vi "Process.vi"(8 "error in":errorcluster, 11 "Instrument.OxfordVRM UI.lvclass":refnum<class "Instrument.OxfordVRM UI.lvclass">) -> (0 "error out":errorcluster, 3 "Instrument.OxfordVRM UI.lvclass":refnum<class "Instrument.OxfordVRM UI.lvclass">)   [LabVIEW 2019, in "Instrument.OxfordVRM UI.lvclass"]
doc: "---------------------------------------------------------------\nJKI State Machine Objects™\nhttp://jki.net/state-machine-objects/\nCopyright (C) 2005-2015, JKI <info@jki.net>\nALL RIGHTS RESERVEDJKI State Machine Objects (SMO) 1.0.0.5\nJKI - JKI\nCopyright (c) 2016, JKI"
uses:
  Instrument.OxfordVRM UI.lvclass
  <vilib>/JKI/JKI SMO/SMO/SMO.lvclass
  <vilib>/JKI/JKI SMO/SMO.UI/SMO.UI.lvclass
  <userlib>/LevyLab/Instrument Framework/Instrument/Instrument.lvclass
  Instrument.OxfordVRM/Typedefs/getAll.ctl
  Instrument.OxfordVRM/Instrument.OxfordVRM.lvclass
  <userlib>/LevyLab/Instrument Framework/Instrument UI/Instrument UI.lvclass
  Instrument.OxfordVRM/Typedefs/VRM Magnet Axis--Enum.ctl
  C:/Program Files (x86)/National Instruments/LabVIEW 2019/user.lib/LevyLab/Instrument Framework/Instrument Types/Cryostat/Instrument.Cryostat.lvclass
  C:/Program Files (x86)/National Instruments/LabVIEW 2019/user.lib/LevyLab/Instrument Framework/Instrument/Instrument.lvclass
  C:/Program Files (x86)/National Instruments/LabVIEW 2019/vi.lib/JKI/JKI SMO/SMO/SMO.lvclass
  C:/Program Files (x86)/National Instruments/LabVIEW 2019/user.lib/LevyLab/Instrument Framework/Instrument UI/Instrument UI.lvclass
  C:/Program Files (x86)/National Instruments/LabVIEW 2019/vi.lib/JKI/JKI SMO/SMO.UI/SMO.UI.lvclass
panel:
  in  "Rate (T/min)":dbl[](array[numeric])=[0.0]
  out "Status":string[](array[string])
  in  "Coordinates":enum16{"XYZ", "Sph"}(ring)
  out "Set Rate (T/min)":dbl[](array[numeric])
  in  "Target (T)":dbl[](array[numeric])=[0.0, 0.0, 0.0]
  out "Setpoint (T)":dbl[](array[numeric])
  out "Field (T)":dbl[](array[numeric])
  out "XY Graph":cluster{dbl[], dbl[]}[](graph)
  out "XZ Graph":cluster{dbl[], dbl[]}[](graph)
  out "Voltage Meter 6":dbl(knob) scale=-10.0..10.0
  out "Voltage Meter 5":dbl(knob) scale=-10.0..10.0
  out "Voltage Meter 4":dbl(knob) scale=-10.0..10.0
  out "Voltage Meter 3":dbl(knob) scale=-10.0..10.0
  out "Voltage Meter 2":dbl(knob) scale=-10.0..10.0
  out "Current Meter 6":dbl(knob) scale=-120.0..120.0
  out "Current Meter 5":dbl(knob) scale=-120.0..120.0
  out "Current Meter 4":dbl(knob) scale=-120.0..120.0
  out "Current Meter 3":dbl(knob) scale=-120.0..120.0
  out "Current Meter 2":dbl(knob) scale=-120.0..120.0
  out "Voltage Meter 1":dbl(knob) scale=-10.0..10.0
  out "Current Meter 1":dbl(knob) scale=-120.0..120.0
  out "System Time (HH:MM:SS)":dbl=165.3592643737793 format="%<%I:%M:%S %p>T"
  out "ETA":dbl=3660699600.0 format="%<%I:%M:%S %p %m/%d/%Y>T"
  out "version":string="v20/10/28"
  in  "Window Maximize":bool
  in  "Window Minimize":bool
  in  "Hold":bool
  in  "To Set":bool
  in  "Export":bool
  in  "To Zero":bool
  in  "Clamp":bool
  out "Magnet Status 2":string="Status: Clamped"
  in  "Power":bool
  # "Status"
  # "x"
  # "Actions"
  # "Targets"
  # "Status"
  # "x"
  # "y"
  # "X \t\t\nCurrent (A)\tField (T)\t    Rate (T/')\n0  - 30 \t   0    - 0.6 \t  0.06\n30 - 42\t    0.6  - 0.85\t  0.048\n42 - 60\t    0.85 - 1.2\t   0.042\n60 - 80\t    1.2  - 1.6\t   0.036\n80 - 99\t    1.6  - 2.0\t   0.024\n\nY \t\t\nCurrent (A)\tField (T)\t    Rate (T/')\n0  - 30\t    0    - 0.6\t   0.048\n30 - 35\t    0.6  - 0.69\t  0.035\n35 - 45\t    0.69 - 0.89\t  0.03\n45 - 60\t    0.89 - 1.2\t   0.024\n60 - 80\t    1.2  - 1.58\t  0.018\n80 - 101\t   1.58 - 2\t     0.01\n\nZ \t\t\nCurrent (A)\tField (T)\t    Rate (T/')\n0  - 30\t    0    - 2.6    0.26\n30 - 60\t    2.6  - 5.3\t   0.21\n60 - 80\t    5.3  - 7.1\t   0.16\n80 - 90\t    7.1  - 8\t     0.13\n90 - 101\t   8    - 9\t     0.1\n\n2 OR MORE AXES\n0.005 T/min"
  # "z"
  # "z"
  # "PS Status"
  # "y"
  # "SMO UI Template"
  # "For instructions on how to use the JKI State Machine Objects, examples and video tutorials, visit:\nhttp://jki.net/state-machine-objects/\n\nJKI State Machine Objects™\nhttp://jki.net/state-machine-objects/\nCopyright (C) 2005-2015, JKI <info@jki.net>\nALL RIGHTS RESERVED"
  # "PSU 6 Voltage (V)"
  # "PSU 5 Voltage (V)"
  # "PSU 4 Voltage (V)"
  # "PSU 3 Voltage (V)"
  # "PSU 2 Voltage (V)"
  # "PSU 6 Current (A)"
  # "PSU 5 Current (A)"
  # "PSU 4 Current (A)"
  # "PSU 3 Current (A)"
  # "PSU 2 Current (A)"
  # "PSU 1 Voltage (V)"
  # "PSU 1 Current (A)"
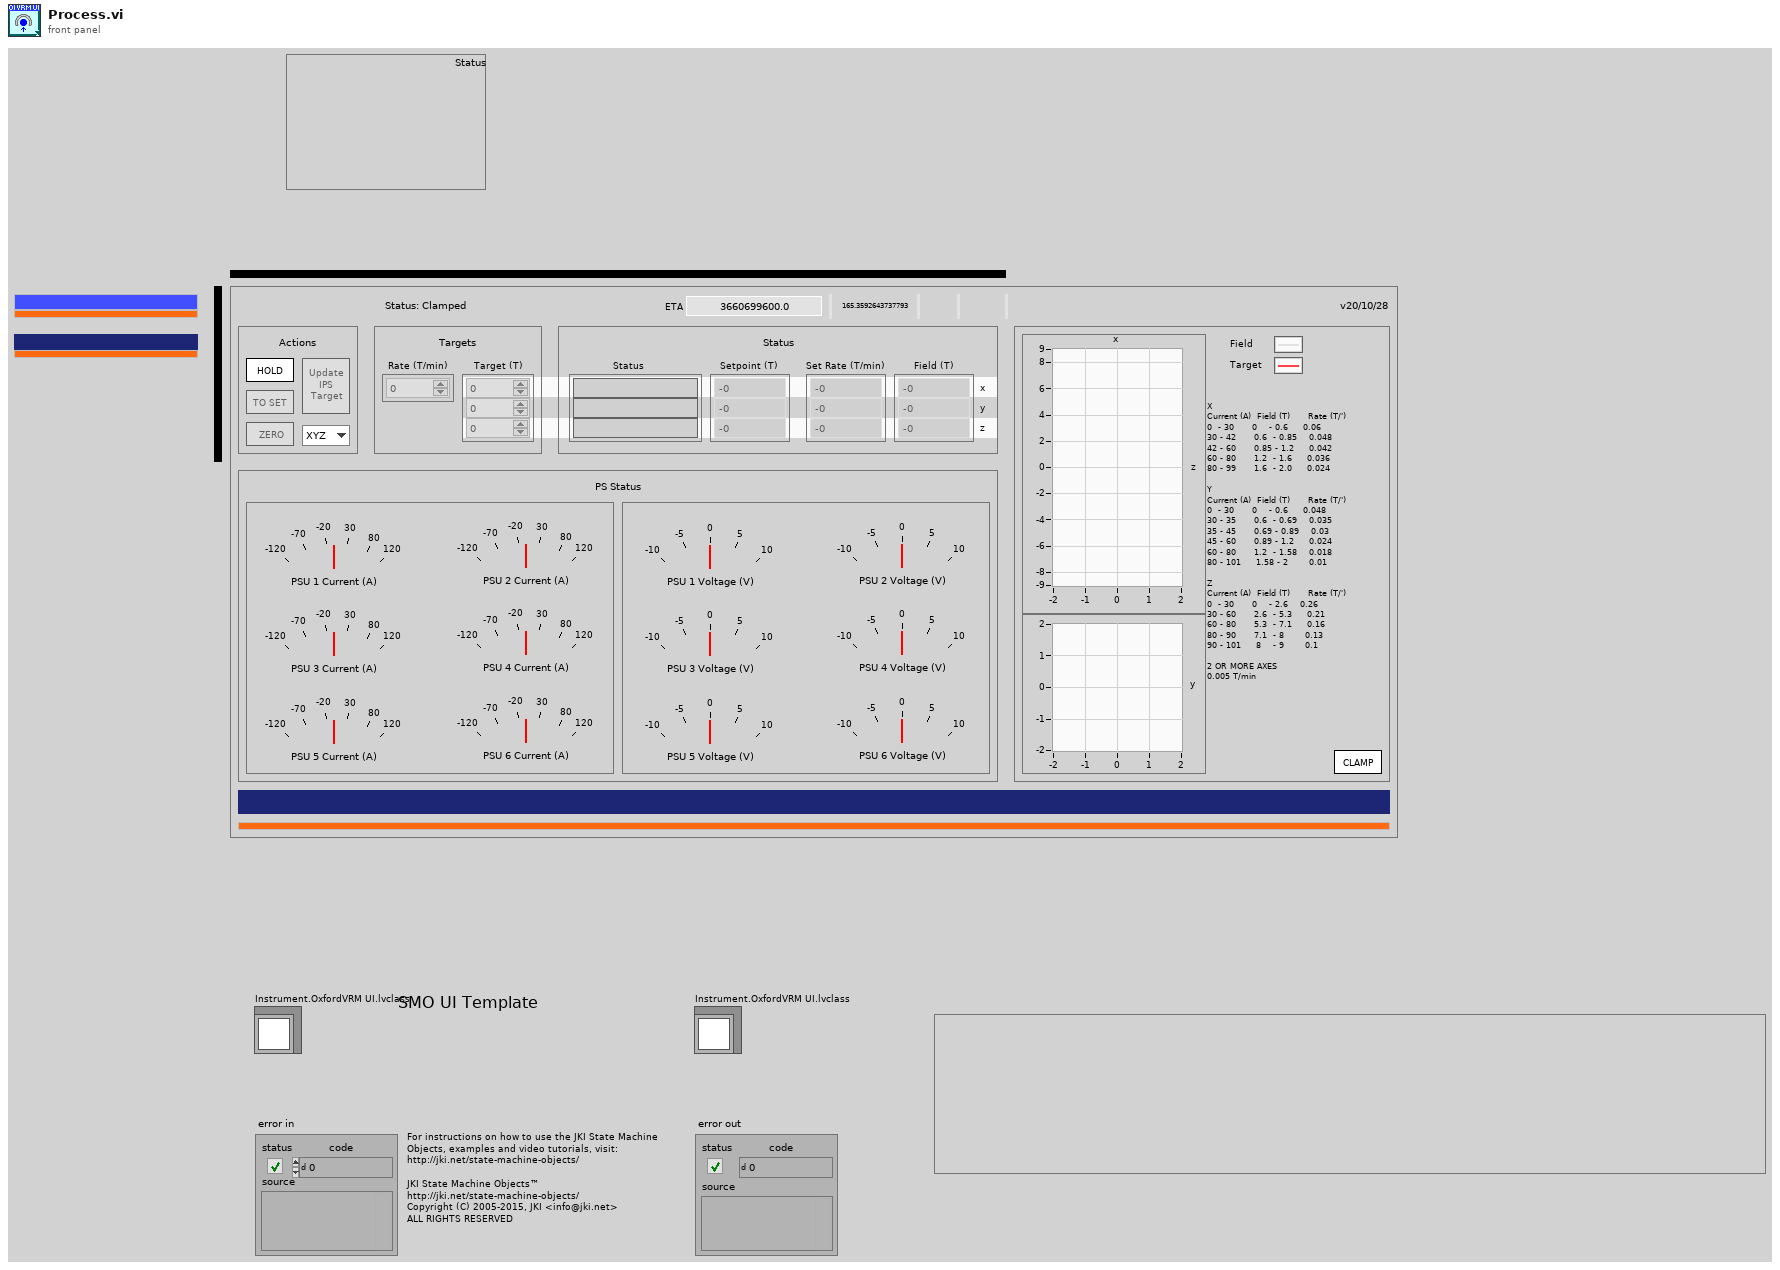
[diagram p1: front panel]
types:
  T1 = typedef "Instrument.OxfordVRM.lvclass/getAll.ctl" = cluster{"Field":dbl[], "Target Field":dbl[], "Target Field Rate":dbl[], "PSU Current":dbl[], "PSU Voltage":dbl[], "Status":string[]}
  T2 = enum32{"invalid app kind", "Development System", "Run Time System", "Student Edition", "Embedded LabVIEW", "Evaluation", "Custom"}
  T3 = enum32{"Invalid", "Standard", "Closed", "Hidden", "Minimized", "Maximized"}
  T4 = typedef "Instrument.OxfordVRM.lvclass/VRM Magnet Axis--Enum.ctl" = enum16{"Z", "X", "Y", "ALL"}
  T5 = cluster{"Core":cluster{"Current VI Reference":refnum<vi>, "Close Panel on Exit?":bool, "error":errorcluster}, "Instrument UI":refnum<class "Instrument.OxfordVRM UI.lvclass">, "Instrument":refnum<class "Instrument.OxfordVRM.lvclass">, "getAll":T1, "Response":string, "config":variant, "Setpoint (XYZ)":dbl[]}
  T6 = typedef "Instrument.OxfordVRM.lvclass/PublicEvents--Instrument.Oxford1820.ProcessStatus.ctl" = string
  T7 = cluster{"Current VI Reference":refnum<vi>, "Close Panel on Exit?":bool, "error":errorcluster}
  T8 = typedef "LVRectTypeDef.ctl" = cluster{"Left":i16, "Top":i16, "Right":i16, "Bottom":i16}
  T9 = typedef "smo.lvlib/SMO.lvclass/Protected Events.ctl" = cluster{"StopProcesses":refnum<user-event>, "AbortProcesses":refnum<user-event>, "Config Changed":refnum<user-event>, "Dependency":refnum<user-event>}
  T10 = typedef "Instrument.lvlib/Instrument.lvclass/PublicEvents--Cluster.ctl" = cluster{"MessageFromProcess":refnum<user-event>}
  T11 = typedef "Instrument.OxfordVRM.lvclass/PublicEvents--Cluster.ctl" = cluster{"ProcessStatus":refnum<user-event>}
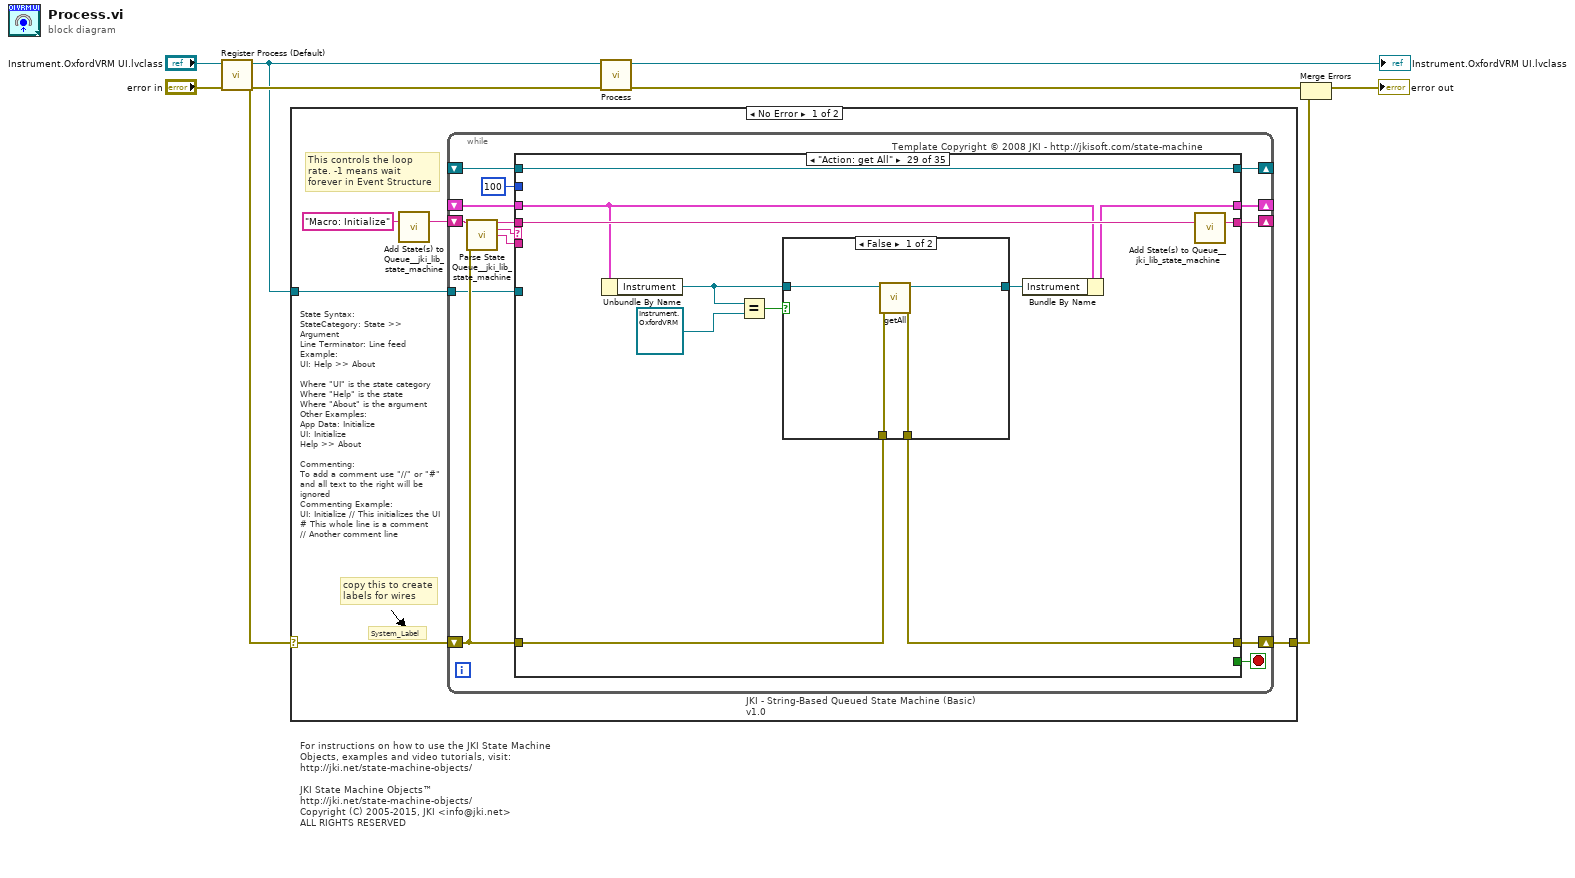
[diagram p0: block diagram]
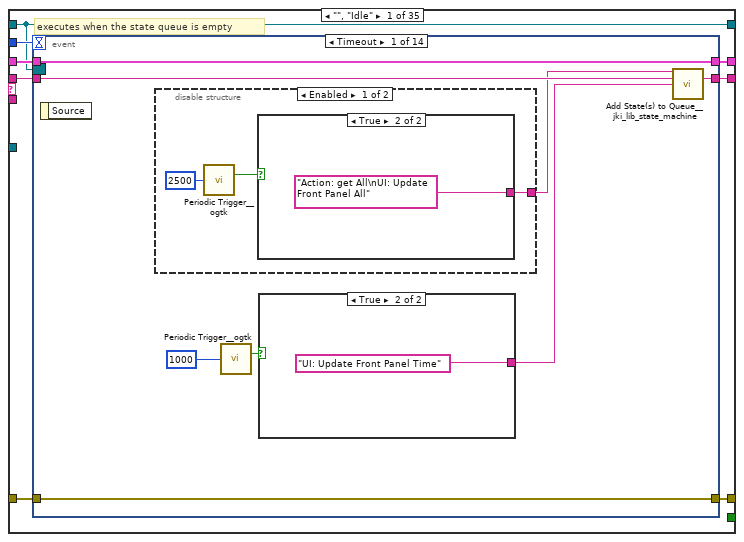
[diagram p2: hidden frame]
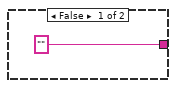
[diagram p3: hidden frame]
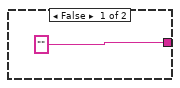
[diagram p4: hidden frame]
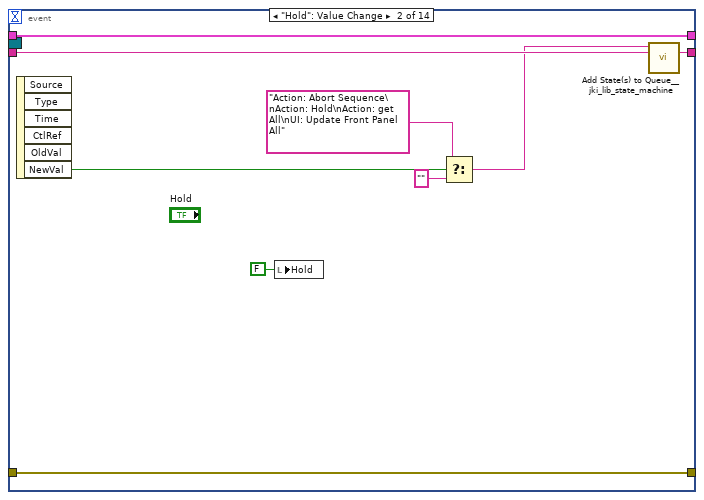
[diagram p6: hidden frame]
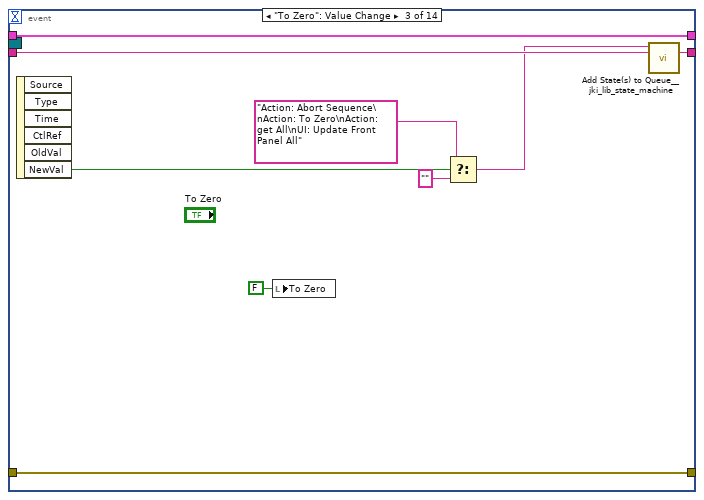
[diagram p7: hidden frame]
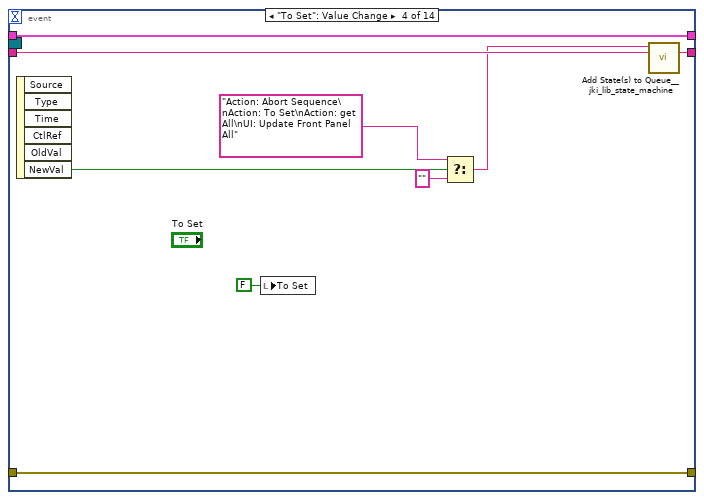
[diagram p8: hidden frame]
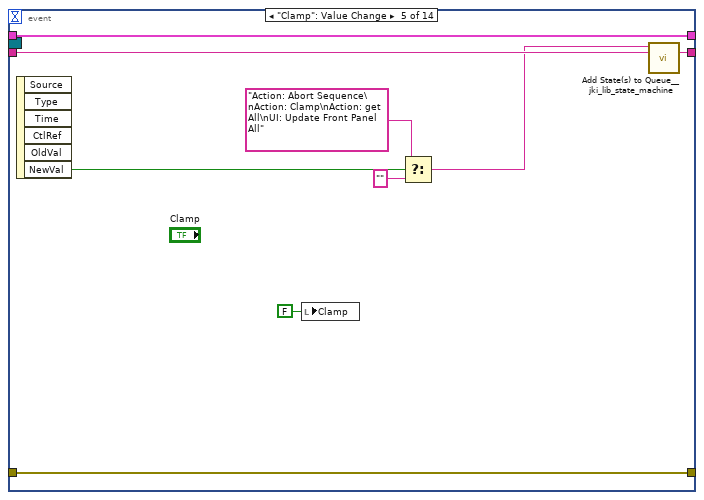
[diagram p9: hidden frame]
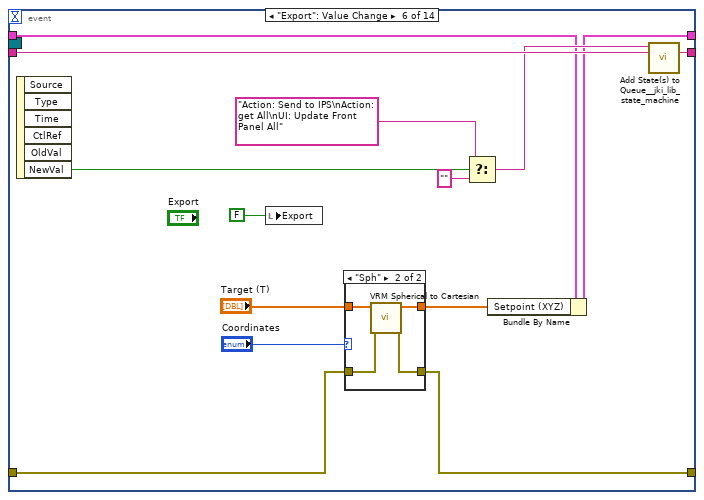
[diagram p10: hidden frame]
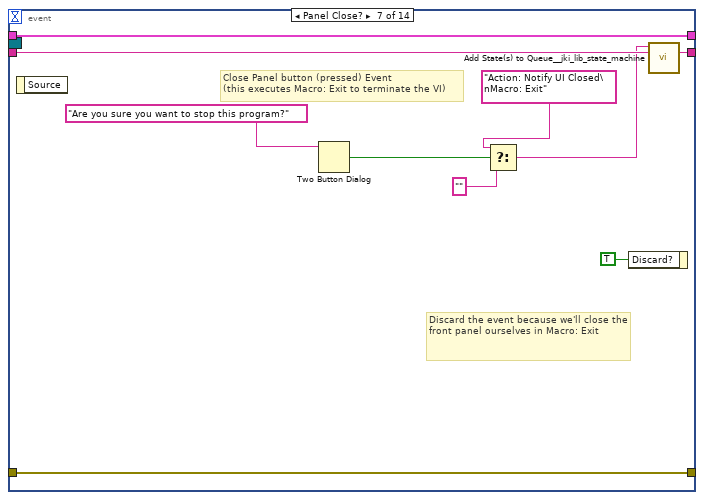
[diagram p12: hidden frame]
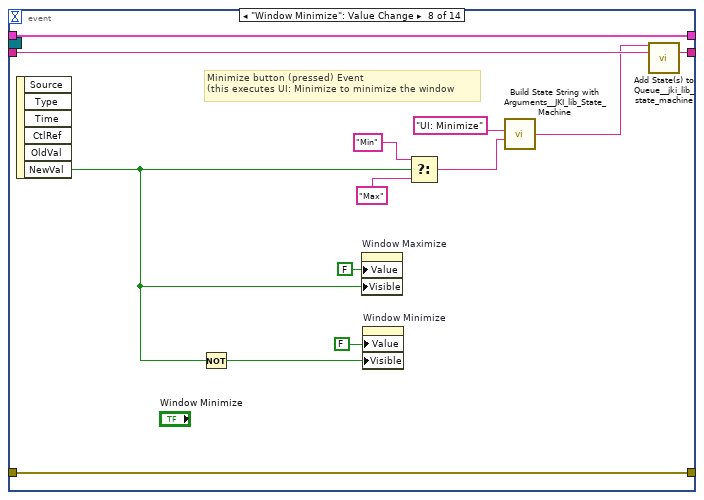
[diagram p13: hidden frame]
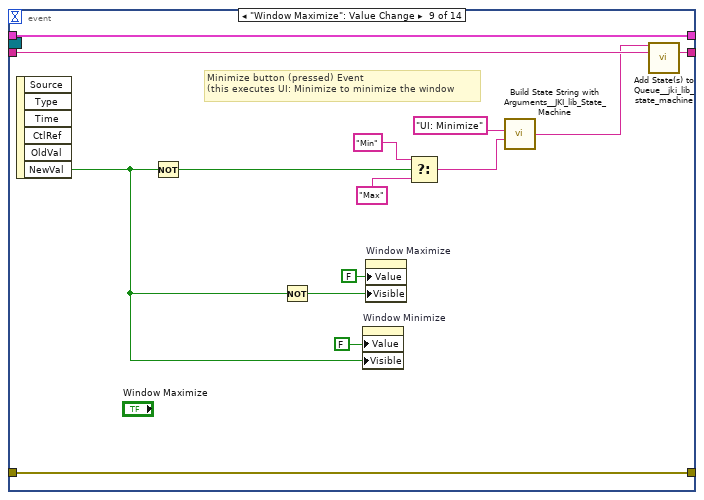
[diagram p14: hidden frame]
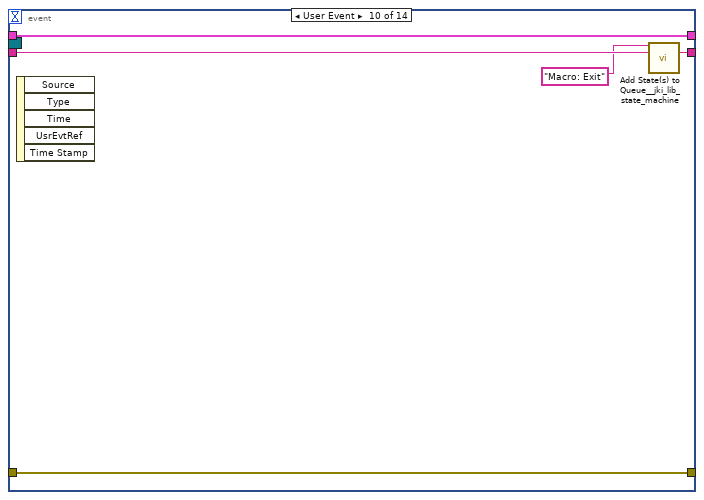
[diagram p15: hidden frame]
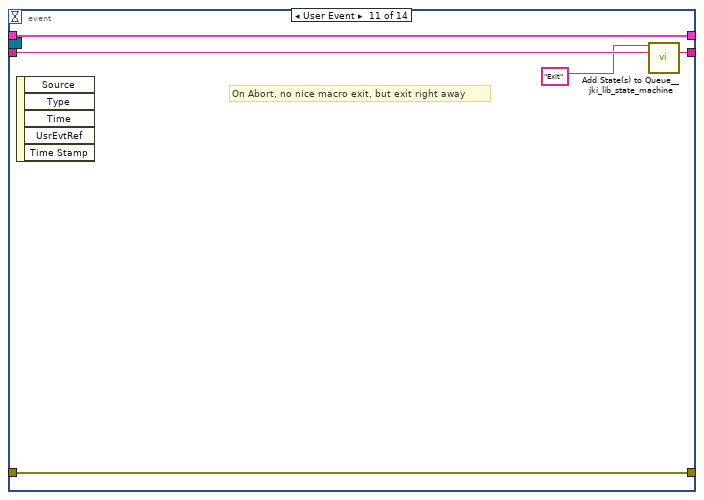
[diagram p16: hidden frame]
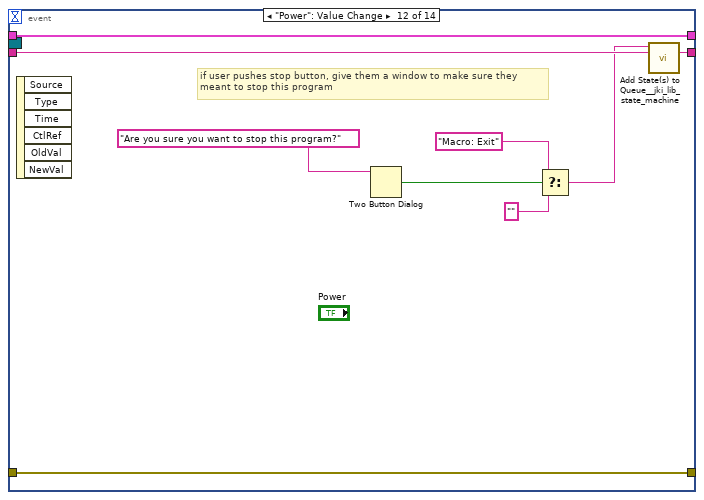
[diagram p17: hidden frame]
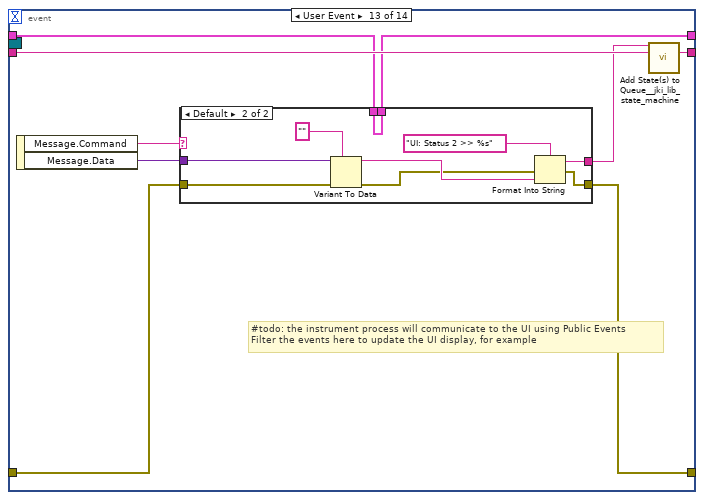
[diagram p18: hidden frame]
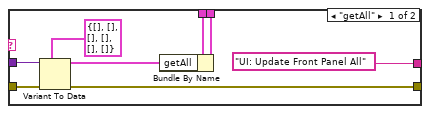
[diagram p19: hidden frame]
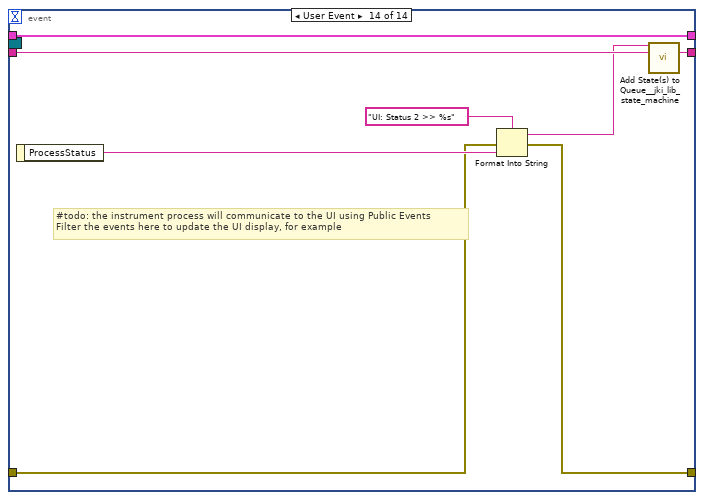
[diagram p20: hidden frame]
diagram:
  # "For instructions on how to use the JKI State Machine Objects, examples and video tutorials, visit:\nhttp://jki.net/state-machine-objects/\n\nJKI State Machine Objects™\nhttp://jki.net/state-machine-objects/\nCopyright (C) 2005-2015, JKI <info@jki.net>\nALL RIGHTS RESERVED"
  n1 = call <vilib>:"Register Process (Default).vi"("error in (no error)"="error in", "SMO"="Instrument.OxfordVRM UI.lvclass") -> ("error out"=w5:errorcluster, "SelfRef"=w4:refnum<class "Instrument.OxfordVRM UI.lvclass">)  [unwired: 8 in]
  n2 = case shown="No Error" w5 {
    selector: w5 -> [w10 w612]
    tunnel: w4 -> [w11 _]
    tunnel: [w9 w612] -> w1
    frame No Error {
      # "State Syntax:\nStateCategory: State >> Argument\nLine Terminator: Line feed\nExample:\nUI: Help >> About\n\nWhere \"UI\" is the state category\nWhere \"Help\" is the state\nWhere \"About\" is the argument\nOther Examples:\nApp Data: Initialize\nUI: Initialize\nHelp >> About\n\nCommenting:\nTo add a comment use \"//\" or \"#\" and all text to the right will be ignored\nCommenting Example:\nUI: Initialize // This initializes the UI\n# This whole line is a comment\n// Another comment line"
      # "copy this to create labels for wires"
      # "This controls the loop rate. -1 means wait forever in Event Structure"
      # "System_Label"
      n3 = call <vilib>:"Add State(s) to Queue__jki_lib_state_machine.vi"("State(s) in (\"\")"="Macro: Initialize") -> ("States Out"=w13:string)  [unwired: 14 in]
      n4 = while "JKI - String-Based Queued State Machine (Basic) v1.0" {
        shift-right: [w20] -> _
        shift-left: _ -> [w19]
        shift-right: [w23] -> w9
        shift-left: w10 -> [w17]
        shift-right: [w22] -> _
        shift-left: w13 -> [w24]
        tunnel: w11 -> [w16]
        shift-right: [w15] -> _
        shift-left: _ -> [w14]
        stop <- w21 stop-if-true
        # "Template Copyright © 2008 JKI - http://jkisoft.com/state-machine"
        n5 = call <vilib>:"Parse State Queue__jki_lib_state_machine.vi"("State Queue"=w24, "Error In (no error)"=w17) -> ("Remaining States"=w26:string, "Current State"=w27:string, "Arguments"=w25:string)  [unwired: 11 in]
        n6 = case shown="\"Action: get All\"" w27 {
          selector: w27 -> [_ _ w203 _ _ _ _ _ _ _ _ _ _ _ _ _ _ _ _ _ _ _ _ _ _ _ _ _ _ _ _ _ _ _ _]
          tunnel: w26 -> [w35 w201 w207 w226 w240 w246 w251 w270 w277 w282 w296 w327 w348 w362 w369 w385 w419 w445 w454 w468 w473 w484 w491 w496 w512 w518 w525 w532 w543 w558 w568 w578 w588 w598 w611]
          tunnel: w25 -> [_ _ _ _ _ _ _ _ _ _ _ _ _ w357 w363 w379 w420 _ _ _ _ _ _ _ _ _ _ _ _ _ _ _ _ _ _]
          tunnel: w19 -> [w33 w198 w205 w217 w228 w242 w248 _ w272 w279 w294 w324 w342 w359 w367 w381 w418 w442 w450 w459 w470 w481 w486 w493 w510 w516 w521 w528 w536 w550 w559 w569 w579 w590 w600]
          tunnel: [w32 w199 w209 w223 w233 w241 w249 w254 w273 w280 w291 w323 w341 w360 w364 w382 w413 w443 w452 w466 w471 w475 w487 w494 w506 w513 w522 w526 w538 w553 w565 w575 w585 w595 w606] -> w23
          tunnel: w17 -> [w31 w199 w208 w223 w229 _ w249 w267 w274 w280 w292 w297 w341 w360 w365 w383 w414 w443 w452 w466 w471 w476 w488 w494 w501 w514 w522 w527 w539 w554 w562 w572 w582 w592 w607]
          tunnel: [w34 w200 w206 w225 w239 w245 w250 w269 w276 w281 w295 w326 w347 w361 w368 w384 w424 w444 w453 w467 w472 w483 w490 w495 w511 w517 w524 w531 w542 w557 w567 w577 w587 w597 w610] -> w22
          tunnel: [_ _ _ _ _ TRUE _ _ _ _ _ _ _ _ _ _ _ _ _ _ _ _ _ _ _ _ _ _ _ _ _ _ _ _ _] -> w21
          tunnel: [w30 w198 w205 w224 w231 w242 w248 w268 w272 w279 w294 w324 w342 w359 w367 w381 w418 w442 w450 w459 w470 w481 w486 w493 w510 w516 w520 w528 w540 w552 w561 w571 w581 w591 w601] -> w20
          tunnel: 100 ("Timeout") -> [w29 _ _ _ _ _ _ _ _ _ _ _ _ _ _ _ _ _ _ _ _ _ _ _ _ _ _ _ _ _ _ _ _ _ _]
          tunnel: w16 -> [_ _ _ _ _ _ _ w261 _ _ _ _ _ _ _ _ _ _ _ _ _ _ _ _ _ _ _ _ _ _ _ _ _ _ _]
          tunnel: [w28 w197 w202 w214 w238 w243 w247 w265 w271 w278 w293 w325 w346 w358 w366 w378 w423 w441 w451 w460 w469 w482 w489 w492 w509 w515 w523 w530 w541 w556 w566 w576 w586 w596 w609] -> w15
          tunnel: w14 -> [w28 w197 w202 w214 w238 w243 w247 w265 w271 w278 w293 w325 w346 w358 w366 w378 w423 w441 w451 w460 w469 w482 w489 w492 _ w515 w523 w530 w541 w556 w566 w576 w586 w596 w609]
          frame "", "Idle" {
            # "executes when the state queue is empty"
            n7 = event shown="[0] Timeout" {
              selector: w28 -> [_ _ _ _ _ _ _ _ _ _ _ _ _ _]
              dyn-events: _ -> [_ _ _ _ _ _ _ _ _ _ _ _ _ _]
              timeout: w29 -> [_ _ _ _ _ _ _ _ _ _ _ _ _ _]
              tunnel: w35 -> [w43 w59 w68 w77 w86 w100 w116 w129 w143 w148 w153 w162 w171 w196]
              tunnel: [w42 w58 w67 w76 w85 w99 w115 w128 w142 w147 w152 w161 w170 w195] -> w34
              tunnel: w33 -> [w39 w56 w65 w74 w83 w93 w113 w127 w141 w145 w150 w159 w169 w190]
              tunnel: [w41 w57 w66 w75 w84 w87 w112 w126 w140 w146 w151 w160 w165 w189] -> w32
              tunnel: w31 -> [w41 w57 w66 w75 w84 w88 w112 w126 w140 w146 w151 w160 w166 w191]
              tunnel: [w39 w56 w65 w74 w83 w92 w113 w127 w141 w145 w150 w159 w168 w190] -> w30
              event Timeout {
                n8 = event-data() -> ()  [unwired: 1 in, 1 out]
                n9 = disable-structure shown="Enabled" {
                  disable-tunnel: [w46 _] -> w40
                  frame Enabled {
                    n10 = call <userlib>:"Periodic Trigger__ogtk.vi"("time (ms)"=u32 2500 ("update time (ms)")) -> ("Triggered"=w48:bool)  [unwired: 12 in, 2 out]
                    n11 = case shown="True" w48 {
                      tunnel: ["" "Action: get All\nUI: Update Front Panel All"] -> w46
                      frame False {
                      }
                      frame True {
                      }
                    }
                  }
                  frame Disabled {
                  }
                }
                n12 = call <userlib>:"Periodic Trigger__ogtk.vi"("time (ms)"=u32 1000 ("update time (ms)")) -> ("Triggered"=w37:bool)  [unwired: 12 in, 2 out]
                n13 = case shown="True" w37 {
                  tunnel: ["" "UI: Update Front Panel Time"] -> w36
                  frame False {
                  }
                  frame True {
                  }
                }
                n14 = call <vilib>:"Add State(s) to Queue__jki_lib_state_machine.vi"("State(s) in Front (\"\")"=w40, "State(s) in (\"\")"=w43, "State(s) at Back (\"\")"=w36) -> ("States Out"=w42:string)  [unwired: 12 in]
              }
              event "Hold": Value Change {
                n15 = event-data() -> ("NewVal"=w55:bool)  [unwired: 1 in, 5 out]
                n16 = local write "Hold"(FALSE ("Hold")) -> ()
                n17 = Select(t="Action: Abort Sequence\nAction: Hold\nAction: get All\nUI: Update Front Panel All" ("State(s) in Front (\"\")"), s=w55, f="") -> (s? t:f=w52:string)
                n18 = call <vilib>:"Add State(s) to Queue__jki_lib_state_machine.vi"("State(s) in Front (\"\")"=w52, "State(s) in (\"\")"=w59) -> ("States Out"=w58:string)  [unwired: 13 in]
              }
              event "To Zero": Value Change {
                n19 = event-data() -> ("NewVal"=w63:bool)  [unwired: 1 in, 5 out]
                n20 = local write "To Zero"(FALSE ("To Zero")) -> ()
                n21 = Select(t="Action: Abort Sequence\nAction: To Zero\nAction: get All\nUI: Update Front Panel All" ("State(s) in Front (\"\")"), s=w63, f="") -> (s? t:f=w61:string)
                n22 = call <vilib>:"Add State(s) to Queue__jki_lib_state_machine.vi"("State(s) in Front (\"\")"=w61, "State(s) in (\"\")"=w68) -> ("States Out"=w67:string)  [unwired: 13 in]
              }
              event "To Set": Value Change {
                n23 = event-data() -> ("NewVal"=w72:bool)  [unwired: 1 in, 5 out]
                n24 = local write "To Set"(FALSE ("To Set")) -> ()
                n25 = Select(t="Action: Abort Sequence\nAction: To Set\nAction: get All\nUI: Update Front Panel All" ("State(s) in Front (\"\")"), s=w72, f="") -> (s? t:f=w71:string)
                n26 = call <vilib>:"Add State(s) to Queue__jki_lib_state_machine.vi"("State(s) in Front (\"\")"=w71, "State(s) in (\"\")"=w77) -> ("States Out"=w76:string)  [unwired: 13 in]
              }
              event "Clamp": Value Change {
                n27 = event-data() -> ("NewVal"=w81:bool)  [unwired: 1 in, 5 out]
                n28 = local write "Clamp"(FALSE ("Clamp")) -> ()
                n29 = Select(t="Action: Abort Sequence\nAction: Clamp\nAction: get All\nUI: Update Front Panel All" ("State(s) in Front (\"\")"), s=w81, f="") -> (s? t:f=w79:string)
                n30 = call <vilib>:"Add State(s) to Queue__jki_lib_state_machine.vi"("State(s) in Front (\"\")"=w79, "State(s) in (\"\")"=w86) -> ("States Out"=w85:string)  [unwired: 13 in]
              }
              event "Export": Value Change {
                n31 = event-data() -> ("NewVal"=w98:bool)  [unwired: 1 in, 5 out]
                n32 = local write "Export"(FALSE ("Send to IPS")) -> ()
                n33 = case shown="\"Sph\"" "Coordinates" {
                  tunnel: "Target (T)" -> [w102 w106]
                  tunnel: [w102 w105] -> w89
                  tunnel: w88 -> [w101 w104]
                  tunnel: [w101 w103] -> w87
                  frame "XYZ", Default {
                  }
                  frame "Sph" {
                    n34 = call "VRM Spherical to Cartesian.vi"("error in (no error)"=w104, "Field (r,theta,phi)"=w106) -> ("error out"=w103:errorcluster, "Field (x,y,z)"=w105:dbl[])  [unwired: 8 in]
                  }
                }
                n35 = Select(t="Action: Send to IPS\nAction: get All\nUI: Update Front Panel All" ("State(s) in Front (\"\")"), s=w98, f="") -> (s? t:f=w95:string)
                n36 = Bundle By Name(cluster=w93, "Setpoint (XYZ)"=w89) -> (w92:T5)
                n37 = call <vilib>:"Add State(s) to Queue__jki_lib_state_machine.vi"("State(s) in Front (\"\")"=w95, "State(s) in (\"\")"=w100) -> ("States Out"=w99:string)  [unwired: 13 in]
              }
              event Panel Close? {
                # "Discard the event because we'll close the front panel ourselves in Macro: Exit"
                # "Close Panel button (pressed) Event\n(this executes Macro: Exit to terminate the VI)"
                n38 = event-data() -> ()  [unwired: 1 in, 1 out]
                n39 = Two Button Dialog(message="Are you sure you want to stop this program?") -> (T button?=w111:bool)  [unwired: 2 in]
                n40 = Select(t="Action: Notify UI Closed\nMacro: Exit", s=w111, f="") -> (s? t:f=w107:string)
                n41 = event-data("Discard?"=TRUE) -> ()  [unwired: 1 in, 1 out]
                n42 = call <vilib>:"Add State(s) to Queue__jki_lib_state_machine.vi"("State(s) in Front (\"\")"=w107, "State(s) in (\"\")"=w116) -> ("States Out"=w115:string)  [unwired: 13 in]
              }
              event "Window Minimize": Value Change {
                # "Minimize button (pressed) Event\n(this executes UI: Minimize to minimize the window"
                n43 = event-data() -> ("NewVal"=w117:bool)  [unwired: 1 in, 5 out]
                n44 = Not(x=w117) -> (.not. x?=w118:bool)
                n45 = property on="Window Maximize" class="Bool (strict)"("Value"=FALSE ("Window Maximize"), "Visible"=w117) -> ()  [unwired: 2 in, 2 out]
                n46 = property on="Window Minimize" class="Bool (strict)"("Value"=FALSE ("Window Maximize"), "Visible"=w118) -> ()  [unwired: 2 in, 2 out]
                n47 = Select(t="Min" ("Arguments (\"\")"), s=w117, f="Max" ("Arguments (\"\")")) -> (s? t:f=w122:string)
                n48 = call <vilib>:"Build State String with Arguments__JKI_lib_State_Machine.vi"("Arguments (\"\")"=w122, "State"="UI: Minimize") -> ("State with Arguments"=w121:string)  [unwired: 4 in]
                n49 = call <vilib>:"Add State(s) to Queue__jki_lib_state_machine.vi"("State(s) in Front (\"\")"=w121, "State(s) in (\"\")"=w129) -> ("States Out"=w128:string)  [unwired: 13 in]
              }
              event "Window Maximize": Value Change {
                # "Minimize button (pressed) Event\n(this executes UI: Minimize to minimize the window"
                n50 = event-data() -> ("NewVal"=w131:bool)  [unwired: 1 in, 5 out]
                n51 = Not(x=w131) -> (.not. x?=w132:bool)
                n52 = Not(x=w131) -> (.not. x?=w130:bool)
                n53 = property on="Window Minimize" class="Bool (strict)"("Value"=FALSE ("Window Maximize"), "Visible"=w131) -> ()  [unwired: 2 in, 2 out]
                n54 = property on="Window Maximize" class="Bool (strict)"("Value"=FALSE ("Window Maximize"), "Visible"=w130) -> ()  [unwired: 2 in, 2 out]
                n55 = Select(t="Min" ("Arguments (\"\")"), s=w132, f="Max" ("Arguments (\"\")")) -> (s? t:f=w136:string)
                n56 = call <vilib>:"Build State String with Arguments__JKI_lib_State_Machine.vi"("Arguments (\"\")"=w136, "State"="UI: Minimize") -> ("State with Arguments"=w135:string)  [unwired: 4 in]
                n57 = call <vilib>:"Add State(s) to Queue__jki_lib_state_machine.vi"("State(s) in Front (\"\")"=w135, "State(s) in (\"\")"=w143) -> ("States Out"=w142:string)  [unwired: 13 in]
              }
              event User Event {
                n58 = event-data() -> ()  [unwired: 1 in, 5 out]
                n59 = call <vilib>:"Add State(s) to Queue__jki_lib_state_machine.vi"("State(s) in Front (\"\")"="Macro: Exit", "State(s) in (\"\")"=w148) -> ("States Out"=w147:string)  [unwired: 13 in]
              }
              event User Event {
                # "On Abort, no nice macro exit, but exit right away"
                n60 = event-data() -> ()  [unwired: 1 in, 5 out]
                n61 = call <vilib>:"Add State(s) to Queue__jki_lib_state_machine.vi"("State(s) in Front (\"\")"="Exit", "State(s) in (\"\")"=w153) -> ("States Out"=w152:string)  [unwired: 13 in]
              }
              event "Power": Value Change {
                # "if user pushes stop button, give them a window to make sure they\nmeant to stop this program"
                n62 = event-data() -> ()  [unwired: 1 in, 6 out]
                n63 = Two Button Dialog(message="Are you sure you want to stop this program?") -> (T button?=w158:bool)  [unwired: 2 in]
                n64 = Select(t="Macro: Exit", s=w158, f="") -> (s? t:f=w154:string)
                n65 = call <vilib>:"Add State(s) to Queue__jki_lib_state_machine.vi"("State(s) in Front (\"\")"=w154, "State(s) in (\"\")"=w162) -> ("States Out"=w161:string)  [unwired: 13 in]
              }
              event User Event {
                # "#todo: the instrument process will communicate to the UI using Public Events\nFilter the events here to update the UI display, for example"
                n66 = event-data() -> ("Message.Command"=w164:string, "Message.Data"=w163:variant)  [unwired: 1 in]
                n67 = case shown="Default" w164 {
                  tunnel: w163 -> [w176 w187]
                  tunnel: w169 -> [w179 w188]
                  tunnel: [w178 w188] -> w168
                  tunnel: ["UI: Update Front Panel All" w184] -> w167
                  tunnel: w166 -> [w175 w181]
                  tunnel: [w174 w180] -> w165
                  frame "getAll" {
                    n68 = Variant To Data(error in=w175, type=T1 {"Field"=[], "Target Field"=[], "Target Field Rate"=[], "PSU Current"=[], "PSU Voltage"=[], "Status"=[]} ("getAll"), Variant=w176) -> (data=w173:T1, error out=w174:errorcluster)
                    n69 = Bundle By Name(cluster=w179, "getAll"=w173) -> (w178:T5)
                  }
                  frame Default {
                    n70 = Variant To Data(error in=w181, type="", Variant=w187) -> (data=w183:string, error out=w182:errorcluster)
                    n71 = Format Into String(format string="UI: Status 2 >> %s", error in=w182, w183) -> (resulting string=w184:string, error out=w180:errorcluster)  [unwired: 1 in]
                  }
                }
                n72 = call <vilib>:"Add State(s) to Queue__jki_lib_state_machine.vi"("State(s) in Front (\"\")"=w167, "State(s) in (\"\")"=w171) -> ("States Out"=w170:string)  [unwired: 13 in]
              }
              event User Event {
                # "#todo: the instrument process will communicate to the UI using Public Events\nFilter the events here to update the UI display, for example"
                n73 = event-data() -> ("ProcessStatus"=w192:T6)  [unwired: 1 in]
                n74 = Format Into String(format string="UI: Status 2 >> %s", error in=w191, w192) -> (resulting string=w194:string, error out=w189:errorcluster)  [unwired: 1 in]
                n75 = call <vilib>:"Add State(s) to Queue__jki_lib_state_machine.vi"("State(s) in Front (\"\")"=w194, "State(s) in (\"\")"=w196) -> ("States Out"=w195:string)  [unwired: 13 in]
              }
            }
          }
          frame "---------- Core ----------" {
            # "Do not put any code in this frame.\n(it is a separator no-op)"
            n76 = call <vilib>:"Add State(s) to Queue__jki_lib_state_machine.vi"("State(s) in (\"\")"=w201) -> ("States Out"=w200:string)  [unwired: 14 in]
          }
          frame Default {
            w212 = 42 items=["No error", "Argument error", "Memory is full", "Out of zone", "End of file", "File already open", "Generic file I/O error", "File not found", "File permission error", "Disk is full", "Duplicate path", "Too many files open", "System feature not enabled", "Resource file not found", "Cannot add resource", "Resource not found", "Image not found", "Image memory error", "Pen does not exist", "Config type invalid", "Config token not found", "Config parse error", "Config memory error", "Bad external code format", "Bad external code offset", "External code not present", "Null window", "Destroy window error", "Null menu", "Print aborted", "Bad print record", "Print driver error", "Windows error during printing", "Memory error during printing", "Print dialog error", "Generic print error", "Invalid device refnum", "Device not found", "Device parameter error", "Device unit error", "Cannot open device", "Device call aborted", "Generic error", "Cancelled by user", "Object ID too low", "Object ID too high", "Object not in heap", "Unknown heap", "Unknown object (invalid DefProc)", "Unknown object (DefProc not in table)", "Message out of range", "Invalid (null) method", "Unknown message", "Manager call not supported", "Bad address", "Network operation in progress", "Network operation timed out", "Connection is busy", "Network attribute not supported", "Network error", "Address in use", "System out of memory", "Connection aborted", "Connection refused", "Not connected", "Already connected", "Connection closed", "Initialization error (interapplication manager)", "Bad occurrence", "Wait on unbound occurrence handler", "Occurrence queue overflow", "Datalog type conflict", "Unused", "Unrecognized type (interapplication manager)", "Memory corrupt", "Failed to make temporary DLL", "Old CIN version", "Drag socket not found", "Failed to load drop-object", "Failed to register OLE object", "Failed to release OLE object", "Format specifier type mismatch", "Unknown format specifier", "Too few format specifiers", "Too many format specifiers", "Scan failed", "Newer CIN version", "Error converting to variant", "Runtime menu error", "Password tampered", "Variant attribute not found", "Incompatible variant data type", "Event data is not available", "Event Store is not present", "Occurrence is not found", "Event Queue is not created", "Event info is not available", "Refnum passed is NULL", "Error retrieving Class GUID", "Error retrieving CoClass GUID", "Error retrieving TypeLib GUID.", "Bad built application magic bytes.", "Specific driver is different from the specific driver associated with the Logical Name.", "There is no session opened to the class driver.", "Max Error", "MAX - Error with config objects", "MAX - Error loading configuration", "MAX - Group not supported"]
            # "Current State"
            # "Do not delete, rename, or modify this frame.\n(this is used to capture unhandled states and typos)"
            # "Handle mistyped state name (developer tool)"
            n77 = Format Into String(format string="Software Exception: Unhandled State \"%s\"." ("message"), error in=w208, w203) -> (resulting string=w211:string, error out=w210:errorcluster)  [unwired: 1 in]
            n78 = call <vilib>:"Error Cluster From Error Code.vi"("show call chain? (False)"=TRUE, "error in (no error)"=w210, "error message (\"\")"=w211, "error code (0)"=w212) -> ("error out"=w209:errorcluster)  [unwired: 5 in]
            n79 = call <vilib>:"Add State(s) to Queue__jki_lib_state_machine.vi"("State(s) in (\"\")"=w207) -> ("States Out"=w206:string)  [unwired: 14 in]
          }
          frame "Initialize Core Data" {
            # "Do not delete, rename, or modify this frame.\n(this is used to determine panel behavior on exit)"
            # "originally closed?"
            # "exe?"
            # "If panel starts closed or is an EXE, then close it when we exit"
            n80 = property class="VI"() -> ("Front Panel.Open"=w222:bool)  [unwired: 2 in, 2 out]
            n81 = property class="App"() -> ("App.Kind"=w221:T2)  [unwired: 2 in, 2 out]
            n82 = control-ref of="Current VI Reference"() -> (w215:refnum<vi>)
            n83 = Not(x=w222) -> (.not. x?=w219:bool)
            n84 = Equal?(x=w221, y=T2."Run Time System" ("Application:Kind")) -> (x = y?=w218:bool)
            n85 = Or(x=w219, y=w218) -> (x .or. y?=w216:bool)
            n86 = Bundle By Name(cluster=w217, "Core.Current VI Reference"=w215, "Core.Close Panel on Exit?"=w216) -> (w224:T5)
            n87 = call <vilib>:"Add State(s) to Queue__jki_lib_state_machine.vi"("State(s) in (\"\")"=w226) -> ("States Out"=w225:string)  [unwired: 14 in]
          }
          frame "Error Handler" {
            w233 = errorcluster {"status"=FALSE, "code"=0, "source"=""}  # No error
            # "Overwrite this method to handle errors and pass to parent if not handled. Parent will fire a public event if the error is not handled up the chain of classes."
            # "Handle any errors here.\nYou can also output any states to clean-up after errors occur"
            n88 = Unbundle By Name(w228) -> ("Instrument UI"=w237:refnum<class "Instrument.OxfordVRM UI.lvclass">)
            n89 = call-dynamic "Handle Error.vi"("Stop on Unhandled Error (T)"=FALSE, "error in"=w229, "SMO"=w237) -> ("handling error"=w227:errorcluster, "Unhandled error"=w232:errorcluster)  [unwired: 6 in, 1 out]
            n90 = Bundle By Name(cluster=w228, "Core.error"=w232) -> (w231:T5)
            n91 = Select(t="Exit", s=w227, f="") -> (s? t:f=w234:string)
            n92 = call <vilib>:"Add State(s) to Queue__jki_lib_state_machine.vi"("State(s) in Front (\"\")"=w234, "State(s) in (\"\")"=w240) -> ("States Out"=w239:string)  [unwired: 13 in]
          }
          frame "Exit" {
            # "Do not put any code in this frame.\n(No errors that occur here will be handled.)"
            n93 = Unbundle By Name(w242) -> ("Core.error"=w241:errorcluster)
            n94 = call <vilib>:"Add State(s) to Queue__jki_lib_state_machine.vi"("State(s) in (\"\")"=w246) -> ("States Out"=w245:string)  [unwired: 14 in]
          }
          frame "---------- Data ----------" {
            # "Do not put any code in this frame.\n(It is a separator no-op. You can make a copy of this frame to create a new Data frame)"
            n95 = call <vilib>:"Add State(s) to Queue__jki_lib_state_machine.vi"("State(s) in (\"\")"=w251) -> ("States Out"=w250:string)  [unwired: 14 in]
          }
          frame "Data: Initialize" {
            w252 = T1 {"Field"=[], "Target Field"=[], "Target Field Rate"=[], "PSU Current"=[], "PSU Voltage"=[], "Status"=[]}  # getAll
            w253 = dbl[] []  # Setpoint (XYZ)
            w255 = refnum<class "Instrument.OxfordVRM.lvclass"> refnum  # Instrument
            w262 = variant  # config
            w263 = ""  # Response
            w264 = T7 {"Current VI Reference"=refnum, "Close Panel on Exit?"=FALSE, "error"={"status"=FALSE, "code"=0, "source"=""}}  # Core
            w266 = refnum<class "Instrument.OxfordVRM UI.lvclass"> refnum  # Self Reference
            # "do not delete - used by framework"
            # "Data names and types of shift register data are defined by this bundle."
            # "Initialize the shift-register data, here.\n(data names are defined by what you wire into the bundle function)"
            n96 = Variant To Data(error in=w267, type=w266, Variant=w261) -> (data=w260:refnum<class "Instrument.OxfordVRM UI.lvclass">, error out=w259:errorcluster)
            n97 = call <userlib>:"Read Instrument.vi"("error in (no error)"=w259, "Instrument UI in"=w260) -> ("error out"=w254:errorcluster, "Instrument"=w256:refnum<class "Instrument.lvclass">, "Instrument UI"=w257:refnum<class "Instrument.OxfordVRM UI.lvclass">)  [unwired: 7 in]
            n98 = To More Specific Class(target class=w255, reference=w256) -> (specific class reference=w258:refnum<class "Instrument.OxfordVRM.lvclass">)  [unwired: 1 in, 1 out]
            n99 = Bundle("Core"=w264, "Instrument UI"=w257, "Instrument"=w258, "getAll"=w252, "Response"=w263, "config"=w262, "Setpoint (XYZ)"=w253) -> (w268:T5)  [unwired: 1 in]
            n100 = call <vilib>:"Add State(s) to Queue__jki_lib_state_machine.vi"("State(s) in (\"\")"=w270) -> ("States Out"=w269:string)  [unwired: 14 in]
          }
          frame "Data: Cleanup" {
            # "Cleanup any data and references, here.\n(this is called automatically, by the Macro: Exit)"
            n101 = Unbundle By Name(w272) -> ("Core.Current VI Reference"=w275:refnum<vi>)
            n102 = Close Reference(reference=w275, error in (no error)=w274) -> (error out=w273:errorcluster)
            n103 = call <vilib>:"Add State(s) to Queue__jki_lib_state_machine.vi"("State(s) in (\"\")"=w277) -> ("States Out"=w276:string)  [unwired: 14 in]
          }
          frame "---------- UI ----------" {
            # "Do not put any code in this frame.\n(It is a separator no-op. You can make a copy of this frame to create a new UI frame)"
            n104 = call <vilib>:"Add State(s) to Queue__jki_lib_state_machine.vi"("State(s) in (\"\")"=w282) -> ("States Out"=w281:string)  [unwired: 14 in]
          }
          frame "UI: Initialize" {
            # "size window to decoration box on front panel"
            # "Initialize the User Interface, here.\n(this is called automatically, by the Macro: Init)"
            n105 = property on="Window Minimize" class="Bool (strict)"("Value"=FALSE ("Window Maximize"), "Visible"=TRUE ("Window Maximize")) -> ()  [unwired: 2 in, 2 out]
            n106 = property on="Window Maximize" class="Bool (strict)"("Value"=FALSE ("Window Maximize"), "Visible"=FALSE ("Window Maximize")) -> ()  [unwired: 2 in, 2 out]
            n107 = invoke on="Power" class="Bool (strict)" method="Reinit To Default"() -> ()  [unwired: 3 in, 3 out]
            n108 = call <userlib>:"Fit VI window to Largest Dec__ogtk.vi"("error in (no error)"=w292, "border spacing (2 px)"=0) -> ("error out"=w291:errorcluster)  [unwired: 4 in, 1 out]
            n109 = call <userlib>:"MGI Get Executable Version.vi"() -> ("Version"=w285:string)  [unwired: 7 in]
            n110 = Format Into String(format string="v%s" ("version"), w285) -> (resulting string=→"version":string)  [unwired: 2 in, 1 out]
            n111 = call <vilib>:"Add State(s) to Queue__jki_lib_state_machine.vi"("State(s) in (\"\")"=w296) -> ("States Out"=w295:string)  [unwired: 14 in]
          }
          frame "UI: Update Front Panel All" {
            n112 = Unbundle By Name(w324) -> ("getAll"=w298:T1)
            n113 = Unbundle By Name(w298) -> ("Field"=w302:dbl[], "Target Field"=w303:dbl[], "Target Field Rate"=→"Set Rate (T/min)":dbl[], "PSU Current"=w305:dbl[], "PSU Voltage"=w306:dbl[], "Status"=w307:string[])
            n114 = Index Array(array=w305) -> (element #1=→"Current Meter 1":dbl, element #2=→"Current Meter 2":dbl, element #3=→"Current Meter 3":dbl, element #4=→"Current Meter 4":dbl, element #5=→"Current Meter 5":dbl, element #6=→"Current Meter 6":dbl)  [unwired: 6 in]
            n115 = Index Array(array=w306) -> (element #1=→"Voltage Meter 1":dbl, element #2=→"Voltage Meter 2":dbl, element #3=→"Voltage Meter 3":dbl, element #4=→"Voltage Meter 4":dbl, element #5=→"Voltage Meter 5":dbl, element #6=→"Voltage Meter 6":dbl)  [unwired: 6 in]
            n116 = for {
              tunnel: [w335] -> w304 mode=indexing
              tunnel: w307 -> [w334] mode=indexing
              n117 = call "Action Status to Text.vi"("PSU Act Stat"=w334) -> ("Status:"=w335:string)
            }
            "Status" <- w304
            n118 = local read "Coordinates"() -> (w301:enum16{"XYZ", "Sph"})
            n119 = case shown="\"Sph\"" w301 {
              tunnel: w303 -> [w329 w333]
              tunnel: w302 -> [w328 w332]
              tunnel: [w328 w331] -> w300
              tunnel: [w329 w330] -> w299
              frame "XYZ", Default {
              }
              frame "Sph" {
                n120 = call "VRM Cartesian to Spherical.vi"("Field (x,y,z)"=w332) -> ("Field (r,theta,phi)"=w331:dbl[])  [unwired: 9 in, 1 out]
                n121 = call "VRM Cartesian to Spherical.vi"("Field (x,y,z)"=w333) -> ("Field (r,theta,phi)"=w330:dbl[])  [unwired: 9 in, 1 out]
              }
            }
            "Field (T)" <- w300
            "Setpoint (T)" <- w299
            n122 = call "VRM Field Graphs.vi"("error in (no error)"=w297, "Target Field (T)"=w303, "Field (T)"=w302) -> ("error out"=w323:errorcluster, "XY Graph"=→"XY Graph":cluster{dbl[], dbl[]}[], "XZ Graph"=→"XZ Graph":cluster{dbl[], dbl[]}[])  [unwired: 6 in]
            n123 = call <vilib>:"Add State(s) to Queue__jki_lib_state_machine.vi"("State(s) in (\"\")"=w327) -> ("States Out"=w326:string)  [unwired: 14 in]
          }
          frame "UI: Update Front Panel Time" {
            n124 = Unbundle By Name(w342) -> ("getAll"=w336:T1)
            n125 = Get Date/Time In Seconds() -> (seconds since 1Jan1904=w345:timestamp)
            n126 = Unbundle By Name(w336) -> ("Target Field"=w337:dbl[], "Field"=w338:dbl[], "Target Field Rate"=w339:dbl[], "Status"=w340:string[])
            n127 = To Double Precision Float(number=w345) -> (double precision float=→"System Time (HH:MM:SS)":dbl)
            n128 = for {
              tunnel: [w355] -> w343 if=w351
              tunnel: w340 -> [w353] mode=indexing
              tunnel: w339 -> [w349] mode=indexing
              tunnel: w338 -> [w354] mode=indexing
              tunnel: w337 -> [w350] mode=indexing
              n129 = Equal?(x=w353, y="RTOS" ("Status")) -> (x = y?=w351:bool)
              n130 = call "Calculate Sweep ETA.vi"("Target Field Rate (T/min)"=w349, "Magnet Field (T)"=w354, "Target Field (T)"=w350) -> ("ETA timestamp"=w356:timestamp)  [unwired: 6 in, 2 out]
              n131 = To Double Precision Float(number=w356) -> (double precision float=w355:dbl)
            }
            "ETA" <- w343
            n132 = call <vilib>:"Add State(s) to Queue__jki_lib_state_machine.vi"("State(s) in (\"\")"=w348) -> ("States Out"=w347:string)  [unwired: 14 in]
          }
          frame "UI: Status 2" {
            n133 = call <vilib>:"Add State(s) to Queue__jki_lib_state_machine.vi"("State(s) in (\"\")"=w362) -> ("States Out"=w361:string)  [unwired: 14 in]
            "Magnet Status 2" <- w357
          }
          frame "UI: Cursor Set" {
            # "Argument"
            n134 = disable-structure shown="Default" {
              disable-tunnel: w365 -> [w370 w373]
              disable-tunnel: [w370 w372] -> w364
              disable-tunnel: w363 -> [_ w371]
              frame condition #0 {
              }
              frame condition #1 (active) {
                n135 = case shown="\"Idle\", Default" w371 {
                  tunnel: w373 -> [w375 w377]
                  tunnel: [w374 w376] -> w372
                  frame "Idle", Default {
                    n136 = call <vilib>:"Unset Busy.vi"("error in (no error)"=w375) -> ("error out"=w374:errorcluster)  [unwired: 10 in]
                  }
                  frame "Busy" {
                    n137 = call <vilib>:"Set Busy.vi"("error in (no error)"=w377) -> ("error out"=w376:errorcluster)  [unwired: 9 in, 1 out]
                  }
                }
              }
            }
            n138 = call <vilib>:"Add State(s) to Queue__jki_lib_state_machine.vi"("State(s) in (\"\")"=w369) -> ("States Out"=w368:string)  [unwired: 14 in]
          }
          frame "UI: Front Panel State" {
            # "Argument"
            # "Set Front Panel Open or Closed\n(Usage: \"UI: Front Panel State >> Open|Close\")"
            n139 = Unbundle By Name(w381) -> ("Core.Current VI Reference"=w380:refnum<vi>)
            n140 = disable-structure shown="Default" {
              disable-tunnel: w383 -> [w389 w412]
              disable-tunnel: [w388 w412] -> w382
              disable-tunnel: w380 -> [w387 _]
              disable-tunnel: w379 -> [w386 _]
              frame condition #0 (active) {
                n141 = case shown="\"Open\", Default" w386 {
                  tunnel: w389 -> [w393 w406]
                  tunnel: [w395 w407] -> w388
                  tunnel: w387 -> [w394 w404]
                  frame "Open", Default {
                    n142 = property class="VI"(reference=w394, error in=w393) -> (reference out=w391:refnum<vi>, error out=w392:errorcluster, "FP.State"=w390:T3)
                    n143 = case shown="\"Closed\"" w390 {
                      tunnel: [w398 w401] -> w395
                      tunnel: w392 -> [w397 w401]
                      tunnel: w391 -> [w396 _]
                      frame "Closed" {
                        n144 = invoke class="VI" method="FP.Open"(reference=w396, error in=w397, "Activate"=TRUE, "State"=T3."Standard") -> (error out=w398:errorcluster)  [unwired: 1 in, 4 out]
                      }
                      frame Default {
                      }
                    }
                  }
                  frame "Close" {
                    n145 = property class="VI"(reference=w404, error in=w406) -> (reference out=w403:refnum<vi>, error out=w405:errorcluster, "FP.State"=w402:T3)
                    n146 = case shown="Default" w402 {
                      tunnel: [w408 w411] -> w407
                      tunnel: w405 -> [w408 w410]
                      tunnel: w403 -> [_ w409]
                      frame "Invalid", "Closed" {
                      }
                      frame Default {
                        n147 = invoke class="VI" method="FP.Close"(reference=w409, error in=w410) -> (error out=w411:errorcluster)  [unwired: 1 in, 2 out]
                      }
                    }
                  }
                }
              }
              frame condition #1 {
              }
            }
            n148 = call <vilib>:"Add State(s) to Queue__jki_lib_state_machine.vi"("State(s) in (\"\")"=w385) -> ("States Out"=w384:string)  [unwired: 14 in]
          }
          frame "UI: Minimize" {
            # "Do not put any code in this frame.\n(It is a separator no-op. You can make a copy of this frame to create a new UI frame)"
            n149 = Unbundle By Name(w418) -> ("Core.Current VI Reference"=w417:refnum<vi>)
            n150 = property class="VI"(reference=w417, error in=w414) -> (reference out=w416:refnum<vi>, error out=w415:errorcluster, "Front Panel.PanelBounds"=w422:T8)
            n151 = case shown="\"Max\"" w420 {
              tunnel: w422 -> [w425 w433]
              tunnel: [w432 w440] -> w421
              frame "Min", Default {
                n152 = Unbundle By Name(w425) -> ("Left"=w431:i16, "Top"=w429:i16)
                n153 = Add(x=i16 776 ("x 6"), y=w431) -> (x+y=w430:i16)
                n154 = Add(x=w429, y=i16 176 ("x 5")) -> (x+y=w428:i16)
                n155 = Bundle By Name(cluster=w425, "Right"=w430, "Bottom"=w428) -> (w432:T8)
              }
              frame "Max" {
                n156 = Unbundle By Name(w433) -> ("Left"=w439:i16, "Top"=w437:i16)
                n157 = Add(x=i16 1168 ("x 8"), y=w439) -> (x+y=w438:i16)
                n158 = Add(x=w437, y=i16 584 ("x 7")) -> (x+y=w436:i16)
                n159 = Bundle By Name(cluster=w433, "Right"=w438, "Bottom"=w436) -> (w440:T8)
              }
            }
            n160 = property class="VI"(reference=w416, error in=w415, "Front Panel.PanelBounds"=w421) -> (error out=w413:errorcluster)  [unwired: 1 out]
            n161 = call <vilib>:"Add State(s) to Queue__jki_lib_state_machine.vi"("State(s) in (\"\")"=w419) -> ("States Out"=w424:string)  [unwired: 14 in]
          }
          frame "---------- Macro ----------" {
            # "Do not put any code in this frame.\n(It is a separator no-op. You can make a copy of this frame to create a new Macro frame)"
            n162 = call <vilib>:"Add State(s) to Queue__jki_lib_state_machine.vi"("State(s) in (\"\")"=w445) -> ("States Out"=w444:string)  [unwired: 14 in]
          }
          frame "Macro: Initialize" {
            w448 = "UI: Initialize\nUI: Front Panel State >> Open\nUI: Status 2 >> ..."  # UI: Initialize UI: Front Panel State >> Open UI: Status 2 >> ...
            # "Initialization Macro\n(This is called once, when the VI starts)"
            n163 = call <vilib>:"Add State(s) to Queue__jki_lib_state_machine.vi"("State(s) in Front (\"\")"="Data: Initialize\nInitialize Core Data\nEvents: Register", "State(s) in (\"\")"="Process: Sync", "State(s) at Back (\"\")"=w448) -> ("States Out"=w447:string)  [unwired: 12 in]
            n164 = call <vilib>:"Add State(s) to Queue__jki_lib_state_machine.vi"("State(s) in Front (\"\")"=w447, "State(s) in (\"\")"=w454) -> ("States Out"=w453:string)  [unwired: 13 in]
          }
          frame "Macro: Exit" {
            # "Exit Macro\n(This is called once, when the VI exits)"
            n165 = Unbundle By Name(w459) -> ("Core.Close Panel on Exit?"=w465:bool)
            n166 = Select(t="UI: Front Panel State >> Close", s=w465, f="") -> (s? t:f=w462:string)
            n167 = call <vilib>:"Add State(s) to Queue__jki_lib_state_machine.vi"("State(s) in Front (\"\")"="Data: Cleanup\nEvents: Unregister\nProcess: Self Terminate", "State(s) in (\"\")"="Process: Sync", "State(s) at Back (\"\")"="Exit") -> ("States Out"=w456:string)  [unwired: 12 in]
            n168 = call <vilib>:"Add State(s) to Queue__jki_lib_state_machine.vi"("State(s) in (\"\")"=w462, "State(s) at Back (\"\")"=w456) -> ("States Out"=w461:string)  [unwired: 13 in]
            n169 = call <vilib>:"Add State(s) to Queue__jki_lib_state_machine.vi"("State(s) in Front (\"\")"=w461, "State(s) in (\"\")"=w468) -> ("States Out"=w467:string)  [unwired: 13 in]
          }
          frame "---------- Process ----------" {
            # "Template Separator\n(You can make a copy of, or modify, this frame)"
            n170 = call <vilib>:"Add State(s) to Queue__jki_lib_state_machine.vi"("State(s) in (\"\")"=w473) -> ("States Out"=w472:string)  [unwired: 14 in]
          }
          frame "Process: Sync" {
            n171 = Unbundle By Name(w481) -> ("Instrument UI"=w477:refnum<class "Instrument.OxfordVRM UI.lvclass">)
            n172 = call <vilib>:"WaitOnProcessSync.vi"("error in (no error)"=w476, "SMO"=w477) -> ("error out"=w475:errorcluster, "Don't run?"=w480:bool)  [unwired: 7 in, 1 out]
            n173 = Select(t="Data: Cleanup\nEvents: Unregister\nExit", s=w480, f="") -> (s? t:f=w474:string)
            n174 = call <vilib>:"Add State(s) to Queue__jki_lib_state_machine.vi"("State(s) in Front (\"\")"=w474, "State(s) in (\"\")"=w484) -> ("States Out"=w483:string)  [unwired: 13 in]
          }
          frame "Process: Self Terminate" {
            n175 = Unbundle By Name(w486) -> ("Instrument UI"=w485:refnum<class "Instrument.OxfordVRM UI.lvclass">)
            n176 = call <vilib>:"SelfTerminate.vi"("error in (no error)"=w488, "SMO in"=w485) -> ("error out"=w487:errorcluster)  [unwired: 8 in, 1 out]
            n177 = call <vilib>:"Add State(s) to Queue__jki_lib_state_machine.vi"("State(s) in (\"\")"=w491) -> ("States Out"=w490:string)  [unwired: 14 in]
          }
          frame "---------- Events ----------" {
            # "Template Separator\n(You can make a copy of, or modify, this frame)"
            n178 = call <vilib>:"Add State(s) to Queue__jki_lib_state_machine.vi"("State(s) in (\"\")"=w496) -> ("States Out"=w495:string)  [unwired: 14 in]
          }
          frame "Events: Register" {
            # "Expand to add\nmore events"
            # "Base Class Protected Events"
            n179 = Unbundle By Name(w510) -> ("Instrument UI"=w504:refnum<class "Instrument.OxfordVRM UI.lvclass">, "Instrument"=w502:refnum<class "Instrument.OxfordVRM.lvclass">)
            n180 = call <vilib>:"GetProtectedEvents.vi"("SMO"=w504) -> ("error out"=w505:errorcluster, "SMO Protected Events"=w508:T9)  [unwired: 8 in, 1 out]
            n181 = call <userlib>:"Instrument.GetPublicEvents.vi"("Instrument"=w502) -> ("error out"=w503:errorcluster, "Instrument Public Events"=w500:T10, "Instrument out"=w499:refnum<class "Instrument.OxfordVRM.lvclass">)  [unwired: 8 in]
            n182 = call "Instrument.OxfordVRM.GetPublicEvents.vi"("Instrument.VRM in"=w499) -> ("error out"=w497:errorcluster, "VRM Public Events"=w498:T11)  [unwired: 8 in, 1 out]
            n183 = register-events(w508, w500, w498) -> (reference out=w509:refnum<event-registration>, error out=w507:errorcluster)  [unwired: 2 in]
            n184 = Merge Errors(w497, w503, w501, w507, w505) -> (w506:errorcluster)
            n185 = call <vilib>:"Add State(s) to Queue__jki_lib_state_machine.vi"("State(s) in (\"\")"=w512) -> ("States Out"=w511:string)  [unwired: 14 in]
          }
          frame "Events: Unregister" {
            n186 = Unregister For Events(event registration refnum=w515, error in=w514) -> (error out=w513:errorcluster)
            n187 = call <vilib>:"Add State(s) to Queue__jki_lib_state_machine.vi"("State(s) in (\"\")"=w518) -> ("States Out"=w517:string)  [unwired: 14 in]
          }
          frame "---------- Action ----------" {
            n188 = Unbundle By Name(w521) -> ("Instrument UI"=w519:refnum<class "Instrument.OxfordVRM UI.lvclass">)
            n189 = Bundle By Name(cluster=w521, "Instrument UI"=w519) -> (w520:T5)
            n190 = call <vilib>:"Add State(s) to Queue__jki_lib_state_machine.vi"("State(s) in (\"\")"=w525) -> ("States Out"=w524:string)  [unwired: 14 in]
          }
          frame "Action: Notify UI Closed" {
            # "Notify that the UI has been closed"
            n191 = Unbundle By Name(w528) -> ("Instrument UI"=w529:refnum<class "Instrument.OxfordVRM UI.lvclass">)
            n192 = call <vilib>:"Hide.vi"("error in (no error)"=w527, "SMO.UI"=w529) -> ("error out"=w526:errorcluster)  [unwired: 8 in, 1 out]
            n193 = call <vilib>:"Add State(s) to Queue__jki_lib_state_machine.vi"("State(s) in (\"\")"=w532) -> ("States Out"=w531:string)  [unwired: 14 in]
          }
          frame "Action: get All" {
            n194 = Unbundle By Name(w536) -> ("Instrument"=w533:refnum<class "Instrument.OxfordVRM.lvclass">)
            n195 = Equal?(x=w533, y=refnum<class "Instrument.OxfordVRM.lvclass"> refnum ("Instrument")) -> (x = y?=w535:bool)
            n196 = case shown="False" w535 {
              tunnel: w539 -> [w545 w548]
              tunnel: [w544 w548] -> w538
              tunnel: [w546 w549] -> w537
              tunnel: w533 -> [w547 w549]
              frame False {
                n197 = call <userlib>:"getAll.vi"("error in (no error)"=w545, "Instrument in"=w547) -> ("error out"=w544:errorcluster, "Instrument out"=w546:refnum<class "Instrument.OxfordVRM.lvclass">)  [unwired: 7 in, 1 out]
              }
              frame True {
              }
            }
            n198 = Bundle By Name(cluster=w536, "Instrument"=w537) -> (w540:T5)
            n199 = call <vilib>:"Add State(s) to Queue__jki_lib_state_machine.vi"("State(s) in (\"\")"=w543) -> ("States Out"=w542:string)  [unwired: 14 in]
          }
          frame "Action: Abort Sequence" {
            n200 = Unbundle By Name(w550) -> ("Instrument"=w555:refnum<class "Instrument.OxfordVRM.lvclass">)
            n201 = call "Instrument.OxfordVRM.AbortSequence.vi"("error in (no error)"=w554, "Instrument.VRM in"=w555) -> ("error out"=w553:errorcluster, "Instrument.VRM out"=w551:refnum<class "Instrument.OxfordVRM.lvclass">)  [unwired: 8 in]
            n202 = Bundle By Name(cluster=w550, "Instrument"=w551) -> (w552:T5)
            n203 = call <vilib>:"Add State(s) to Queue__jki_lib_state_machine.vi"("State(s) in (\"\")"=w558) -> ("States Out"=w557:string)  [unwired: 14 in]
          }
          frame "Action: Hold" {
            n204 = Unbundle By Name(w559) -> ("Instrument"=w564:refnum<class "Instrument.OxfordVRM.lvclass">)
            n205 = call "Hold.vi"("Axis"=VRM_Magnet_Axis--Enum."ALL", "error in (no error)"=w562, "Instrument.VRM in"=w564) -> ("error out"=w565:errorcluster, "Instrument.VRM out"=w560:refnum<class "Instrument.OxfordVRM.lvclass">)  [unwired: 6 in, 1 out]
            n206 = Bundle By Name(cluster=w559, "Instrument"=w560) -> (w561:T5)
            n207 = call <vilib>:"Add State(s) to Queue__jki_lib_state_machine.vi"("State(s) in (\"\")"=w568) -> ("States Out"=w567:string)  [unwired: 14 in]
          }
          frame "Action: To Zero" {
            n208 = Unbundle By Name(w569) -> ("Instrument"=w573:refnum<class "Instrument.OxfordVRM.lvclass">)
            n209 = call "Ramp to Zero.vi"("Axis"=VRM_Magnet_Axis--Enum."ALL", "error in (no error)"=w572, "Instrument.VRM in"=w573) -> ("error out"=w575:errorcluster, "Instrument.VRM out"=w570:refnum<class "Instrument.OxfordVRM.lvclass">)  [unwired: 6 in, 1 out]
            n210 = Bundle By Name(cluster=w569, "Instrument"=w570) -> (w571:T5)
            n211 = call <vilib>:"Add State(s) to Queue__jki_lib_state_machine.vi"("State(s) in (\"\")"=w578) -> ("States Out"=w577:string)  [unwired: 14 in]
          }
          frame "Action: To Set" {
            n212 = Unbundle By Name(w579) -> ("Instrument"=w583:refnum<class "Instrument.OxfordVRM.lvclass">)
            n213 = call "Ramp to Set.vi"("Axis"=VRM_Magnet_Axis--Enum."ALL", "error in (no error)"=w582, "Instrument.VRM in"=w583) -> ("error out"=w585:errorcluster, "Instrument.VRM out"=w580:refnum<class "Instrument.OxfordVRM.lvclass">)  [unwired: 6 in, 1 out]
            n214 = Bundle By Name(cluster=w579, "Instrument"=w580) -> (w581:T5)
            n215 = call <vilib>:"Add State(s) to Queue__jki_lib_state_machine.vi"("State(s) in (\"\")"=w588) -> ("States Out"=w587:string)  [unwired: 14 in]
          }
          frame "Action: Clamp" {
            n216 = Unbundle By Name(w590) -> ("Instrument"=w593:refnum<class "Instrument.OxfordVRM.lvclass">)
            n217 = call "Clamp.vi"("Axis"=VRM_Magnet_Axis--Enum."ALL", "error in (no error)"=w592, "Instrument.VRM in"=w593) -> ("error out"=w595:errorcluster, "Instrument.VRM out"=w589:refnum<class "Instrument.OxfordVRM.lvclass">)  [unwired: 6 in, 1 out]
            n218 = Bundle By Name(cluster=w590, "Instrument"=w589) -> (w591:T5)
            n219 = call <vilib>:"Add State(s) to Queue__jki_lib_state_machine.vi"("State(s) in (\"\")"=w598) -> ("States Out"=w597:string)  [unwired: 14 in]
          }
          frame "Action: Send to IPS" {
            n220 = Unbundle By Name(w600) -> ("Instrument"=w608:refnum<class "Instrument.OxfordVRM.lvclass">, "Setpoint (XYZ)"=w602:dbl[])
            n221 = Index Array(array="Rate (T/min)") -> (element=w604:dbl)  [unwired: 1 in]
            n222 = call "Set Target.vi"("Axis"=VRM_Magnet_Axis--Enum."ALL", "error in (no error)"=w607, "Target Rate Limit (T/min)"=w604, "Target Field (T)"=w602, "Instrument.VRM in"=w608) -> ("error out"=w606:errorcluster, "Instrument.VRM out"=w599:refnum<class "Instrument.OxfordVRM.lvclass">)  [unwired: 4 in, 1 out]
            n223 = Bundle By Name(cluster=w600, "Instrument"=w599) -> (w601:T5)
            n224 = call <vilib>:"Add State(s) to Queue__jki_lib_state_machine.vi"("State(s) in (\"\")"=w611) -> ("States Out"=w610:string)  [unwired: 14 in]
          }
        }
      }
    }
    frame Error {
    }
  }
  n225 = call-parent "Process.vi"("error in"=w5, "Instrument UI in"=w4) -> ("error out"=w2:errorcluster, "Instrument UI out"=→"Instrument.OxfordVRM UI.lvclass":refnum<class "Instrument.OxfordVRM UI.lvclass">)  [unwired: 8 in]
  n226 = Merge Errors(w2, w1) -> (→"error out":errorcluster)
